vi "OBIS Laser Info.vi"() -> ()   [LabVIEW 8.6]
uses:
  <vilib>/Instr/_visa.llb/VISA Configure Serial Port (Instr).vi
panel:
  out "Laser Hours":string
  out "Wavelength":string
  out "Laser Model":string
  out "Serial Number":string
  in  "VISA resource name":refnum<visa-resource-name>
  # "Select the appropriate VISA resource name (COM port number) for the laser and run this VI to gather information about the laser."
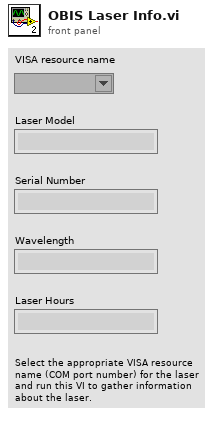
[diagram p1: front panel]
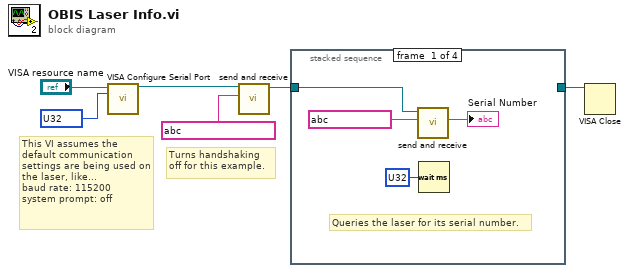
[diagram p0: block diagram]
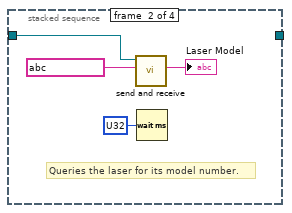
[diagram p2: hidden frame]
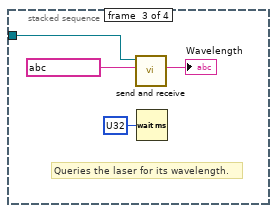
[diagram p3: hidden frame]
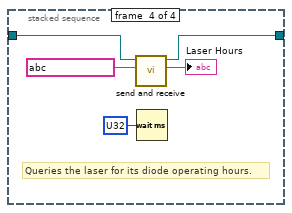
[diagram p4: hidden frame]
diagram:
  # "Turns handshaking\noff for this example."
  # "This VI assumes the default communication settings are being used on the laser, like...\nbaud rate: 115200\nsystem prompt: off"
  n1 = call-poly "VISA Configure Serial Port"("VISA resource name"="VISA resource name", "baud rate (9600)"=u32 ?) -> ("VISA resource name out"=w3:refnum<visa-resource-name>)  [unwired: 12 in, 1 out]
  n2 = call "send and receive.vi"("write to laser"=string ?, "VISA resource name"=w3) -> ("VISA resource name out"=w2:refnum<visa-resource-name>)  [unwired: 8 in, 1 out]
  n3 = stacked-sequence {
    tunnel: w2 -> [w9 w13 w17 w22]
    tunnel: [_ _ _ w19] -> w4
    frame #0 {
      # "Queries the laser for its serial number."
      n4 = call "send and receive.vi"("write to laser"=string ?, "VISA resource name"=w9) -> ("read from laser"=→"Serial Number":string)  [unwired: 8 in, 1 out]
      n5 = Wait (ms)(milliseconds to wait=u32 ?) -> ()  [unwired: 1 out]
    }
    frame #1 {
      # "Queries the laser for its model number."
      n6 = call "send and receive.vi"("write to laser"=string ?, "VISA resource name"=w13) -> ("read from laser"=→"Laser Model":string)  [unwired: 8 in, 1 out]
      n7 = Wait (ms)(milliseconds to wait=u32 ?) -> ()  [unwired: 1 out]
    }
    frame #2 {
      # "Queries the laser for its wavelength."
      n8 = call "send and receive.vi"("write to laser"=string ?, "VISA resource name"=w17) -> ("read from laser"=→"Wavelength":string)  [unwired: 8 in, 1 out]
      n9 = Wait (ms)(milliseconds to wait=u32 ?) -> ()  [unwired: 1 out]
    }
    frame #3 {
      # "Queries the laser for its diode operating hours."
      n10 = call "send and receive.vi"("write to laser"=string ?, "VISA resource name"=w22) -> ("read from laser"=→"Laser Hours":string, "VISA resource name out"=w19:refnum<visa-resource-name>)  [unwired: 8 in]
      n11 = Wait (ms)(milliseconds to wait=u32 ?) -> ()  [unwired: 1 out]
    }
  }
  n12 = VISA Close(VISA resource name=w4) -> ()  [unwired: 1 in, 1 out]
